vi "Destroy.vi"(8 "Error In":errorcluster, 11 "Session":refnum<class "Session.lvclass">) -> (0 "Error Out":errorcluster, 3 "SSH":refnum<class "SSH.lvclass">)   [LabVIEW 2018, in "Toolkit.lvlib" / "Session.lvclass"]
doc: "Cleanly and safely free the session in underlying libssh2 shared library. This must be called, or executed, after all other session-related VIs. Once this is called, no other session-related VIs should be called, or executed. This frees all internal memory used by the libssh2 shared library for this session and a segmentation fault will occur if session-related VIs are executed for this session object."
uses:
  Session.lvclass
  SSH/SSH.lvclass
  Session.lvclass/Session.ctl
  SSH/SSH.lvclass/SSH.ctl
  Toolkit.lvlib
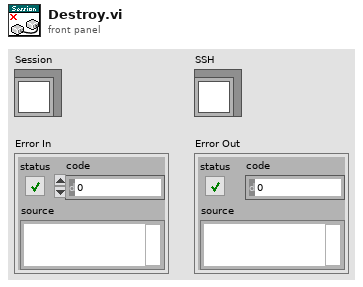
[diagram p1: front panel]
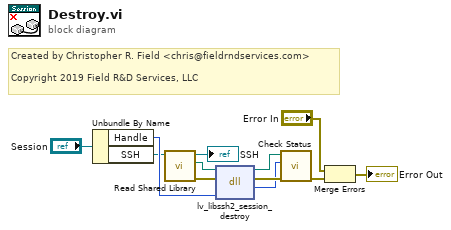
[diagram p0: block diagram]
diagram:
  # "Created by Christopher R. Field <chris@fieldrndservices.com>\n\nCopyright 2019 Field R&D Services, LLC"
  n1 = Unbundle By Name("Session") -> ("Handle"=w10:u64, "SSH"=w4:refnum<class "SSH.lvclass">)
  n2 = call "Read Shared Library.vi"("SSH In"=w4) -> ("Error Out"=w1:errorcluster, "libssh2lv Shared Library"=w2:path, "SSH Out"=→"SSH":refnum<class "SSH.lvclass">)  [unwired: 8 in]
  n3 = dll-call lib="D:/Users/cfield/Code/Field R&D Services/SSH/LV-LIBSSH2/LabVIEW/trunk/src/Toolkit/Support/lv-libssh2.dll" fn="lv_libssh2_session_destroy"(path in=w2, error in=w1, "handle"=w10) -> (path out=w7:path, error out=w8:errorcluster, "status"=w5:i32)  [unwired: 2 in]
  n4 = call "Check Status.vi"("Error In"=w8, "Status"=w5, "libssh2lv Shared Library In"=w7) -> ("Error Out"=w6:errorcluster)  [unwired: 7 in, 1 out]
  n5 = Merge Errors("Error In", w6) -> (→"Error Out":errorcluster)
